vi "Set Direction.vi"(8 "error in (no error)":errorcluster, 9 "Interlock Chain":refnum<class "Interlock Chain.lvclass">, 10 "Direction (Down)":enum16{"UP", "DOWN"}(ring)=enum."DOWN", 11 "Cylinder in":refnum<class "Cylinder.lvclass">) -> (0 "error out":errorcluster, 3 "Cylinder out":refnum<class "Cylinder.lvclass">)   [LabVIEW 2015, in "cRIO-Carbondioxide.lvlib" / "CO2-Actor.lvlib" / "Cylinder.lvclass"]
uses:
  Cylinder.lvclass
  Interlocks/Interlock Chain/Interlock Chain.lvclass
  Cylinder.lvclass/Cylinder.ctl
  Valve Messages/Write Bit Field Msg/Write Bit Field Msg.lvclass/Write Bit Field Msg.ctl
  <vilib>/ActorFramework/Message Enqueuer/Message Enqueuer.lvclass/Message Enqueuer.ctl
  <vilib>/ActorFramework/Message Enqueuer/Enqueue.vi
  <vilib>/ActorFramework/Message Priority Queue/Priority Enqueue.vi
  Valve Messages/Write Bit Field Msg/Write Bit Field Msg.lvclass
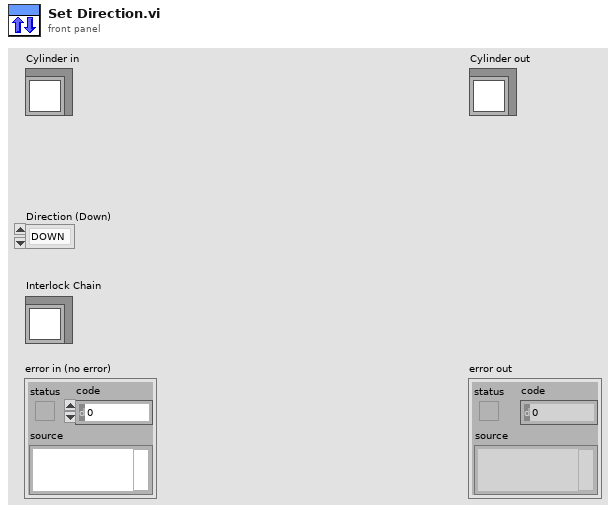
[diagram p1: front panel]
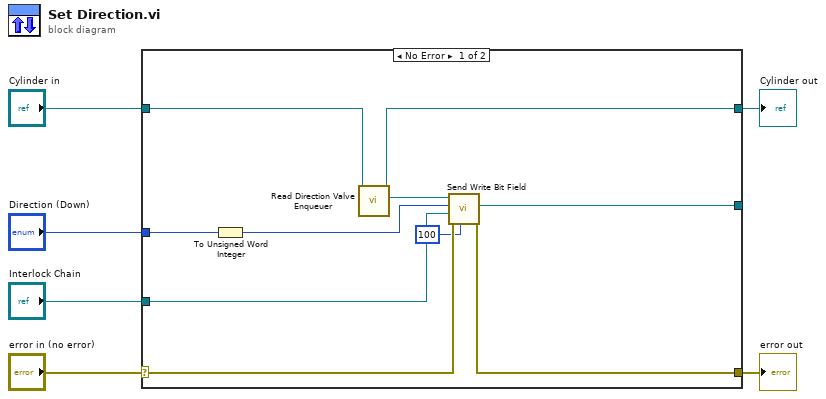
[diagram p0: block diagram]
diagram:
  n1 = case shown="No Error" "error in (no error)" {
    selector: "error in (no error)" -> [w13 w18]
    tunnel: [w12 w18] -> w5
    tunnel: [w10 w17] -> w3
    tunnel: "Cylinder in" -> [w11 w17]
    tunnel: "Direction (Down)" -> [w15 _]
    tunnel: "Interlock Chain" -> [w9 _]
    tunnel: [w7 _] -> _
    frame No Error {
      n2 = To Unsigned Word Integer(number=w15) -> (unsigned 16bit integer=w14:u16)
      n3 = call "Read Direction Valve Enqueuer.vi"("Cylinder in"=w11) -> ("Actor Framework:Message Enqueuer"=w16:refnum<class "Message Enqueuer.lvclass">, "Cylinder out"=w10:refnum<class "Cylinder.lvclass">)  [unwired: 9 in]
      n4 = call "Send Write Bit Field.vi"("Success timeout (0 = dont wait)"=100, "error in (no error)"=w13, "Interlock Chain"=w9, "Bit Field"=w14, "Message Enqueuer"=w16) -> ("error out"=w12:errorcluster, "occurrence"=w7:refnum<k4>)  [unwired: 3 in, 2 out]
    }
    frame Error {
    }
  }
  "error out" <- w5
  "Cylinder out" <- w3
